vi "Get AIs.vi"() -> ()   [LabVIEW 2019]
panel:
  out "output cluster":T1
  in  "Next":bool
  in  "stop":bool
  in  "cRIO IP":string="//172.22.11.2"
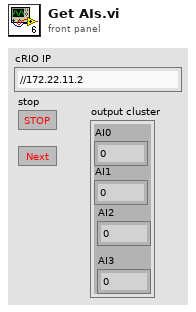
[diagram p1: front panel]
types:
  T1 = cluster{"AI0":dbl, "AI1":dbl, "AI2":dbl, "AI3":dbl}
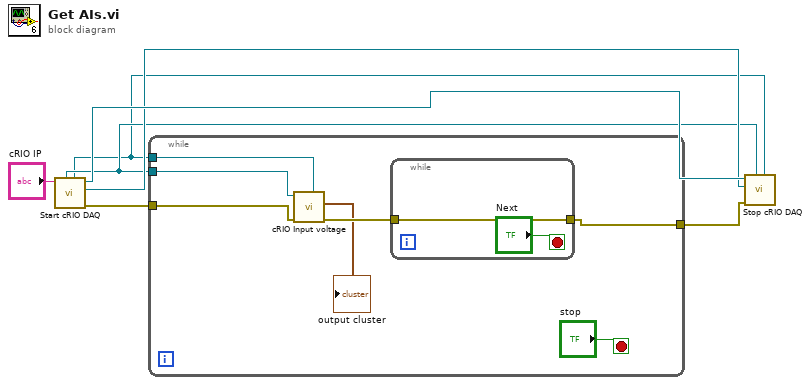
[diagram p0: block diagram]
diagram:
  n1 = call "Start cRIO DAQ.vi"("cRIO IP"="cRIO IP") -> ("error out"=w6:errorcluster, "vi reference"=w4:refnum<vi>, "application reference"=w5:refnum<vi>, "DAQ_AI_Reader endpoint"=w1:refnum<k21>, "DAQ_CMD_Writer endpoint"=w2:refnum<k21>)  [unwired: 6 in]
  n2 = while {
    tunnel: w2 -> [w13]
    tunnel: w1 -> [w12]
    tunnel: w6 -> [w11]
    tunnel: [w10] -> w3
    stop <- "stop" stop-if-true
    n3 = call "cRIO Input voltage.vi"("DAQ_AI_Reader endpoint"=w12, "error in (no error)"=w11, "DAQ_CMD_Writer endpoint"=w13) -> ("error out"=w9:errorcluster, "output cluster"=→"output cluster":T1)  [unwired: 6 in, 1 out]
    n4 = while {
      tunnel: [w16] -> w10
      tunnel: w9 -> [w16]
      stop <- "Next" stop-if-true
    }
  }
  n5 = call "Stop cRIO DAQ.vi"("DAQ_AI_Reader endpoint"=w1, "DAQ_CMD_Writer endpoint"=w2, "error in (no error)"=w3, "VI reference"=w4, "application reference"=w5) -> ()  [unwired: 6 in, 1 out]
